vi "niRFUtil MT UTIL Integer Rate Interpolation.vi"   [LabVIEW 2015, in "niRFUtil.lvlib"]
uses:
  niRFUtil.lvlib
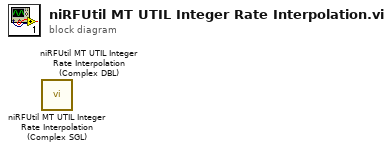
[diagram p0: block diagram]
diagram:
  n1 = call "niRFUtil MT UTIL Integer Rate Interpolation (Complex SGL).vi"() -> ()  [unwired: 10 in, 2 out]
  n2 = call "niRFUtil MT UTIL Integer Rate Interpolation (Complex DBL).vi"() -> ()  [unwired: 10 in, 2 out]
